vi "转换簇到二维数组_new.vi"(11 "Port 0":T1) -> (3 "output 2D array":dbl[][](array[numeric]))   [LabVIEW 2021]
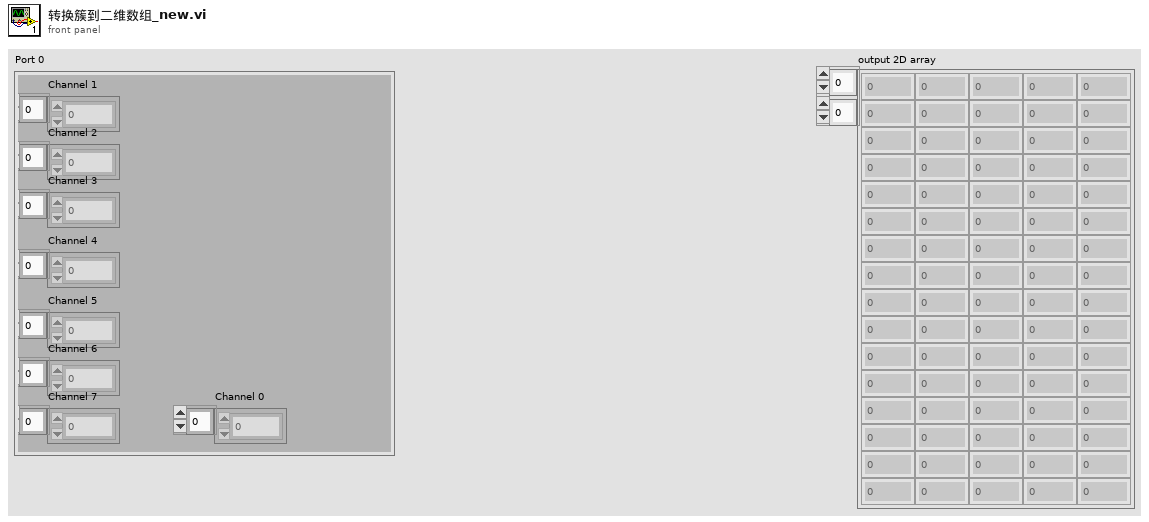
[diagram p1: front panel]
types:
  T1 = cluster{"Channel 1":dbl[], "Channel 2":dbl[], "Channel 3":dbl[], "Channel 4":dbl[], "Channel 5":dbl[], "Channel 6":dbl[], "Channel 7":dbl[], "Channel 0":dbl[]}
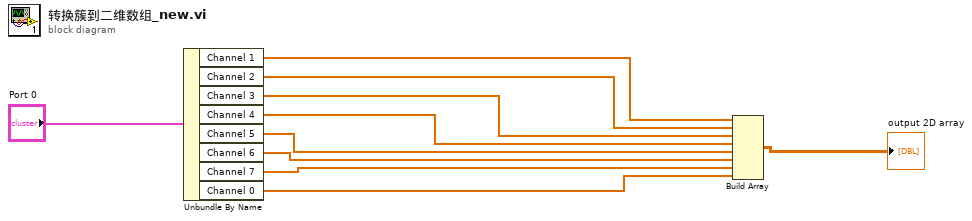
[diagram p0: block diagram]
diagram:
  n1 = Unbundle By Name("Port 0") -> ("Channel 1"=w9:dbl[], "Channel 2"=w1:dbl[], "Channel 3"=w8:dbl[], "Channel 4"=w7:dbl[], "Channel 5"=w6:dbl[], "Channel 6"=w5:dbl[], "Channel 7"=w4:dbl[], "Channel 0"=w3:dbl[])
  n2 = Build Array(w9, w1, w8, w7, w6, w5, w4, w3) -> (→"output 2D array":dbl[][])
